vi "Actor Core.vi"(8 "error in":errorcluster, 11 "Timer in":refnum<class "Timer.lvclass">) -> (0 "error out":errorcluster, 3 "Actor out":refnum<class "Actor.lvclass">)   [LabVIEW 2023, in "Timer.lvlib" / "Timer.lvclass"]
doc: "(<B>Filename</B>: Actor Framework.lvlib:Actor.lvclass:Actor Core.vi)\n\nReceives messages to the actor, reacts to them, and initiates any error handling that may shut the actor down.\n\nDescendant classes may override this VI to append parallel tasks for the actor to complete while it handles messages. Overrides use the Call Parent Class Method node."
uses:
  Timer.lvclass
  C:/Program Files/National Instruments/LabVIEW 2023/vi.lib/ActorFramework/Actor/Actor.lvclass
  <vilib>/ActorFramework/Actor/Actor.lvclass
  Timer.lvclass/Timer.ctl
  <vilib>/ActorFramework/Message Enqueuer/Message Priority.ctl
  <vilib>/ActorFramework/Actor/Actor.lvclass/Actor.ctl
  <vilib>/ActorFramework/Message Enqueuer/Message Enqueuer.lvclass/Message Enqueuer.ctl
  <vilib>/ActorFramework/Message Enqueuer/Init from Existing Queue.vi
  <vilib>/ActorFramework/Message Enqueuer/Enqueue.vi
  Timer Messages/Abort Msg/Abort Msg.lvclass
  C:/Program Files/National Instruments/LabVIEW 2023/vi.lib/ActorFramework/Message/Message.lvclass
  <vilib>/ActorFramework/Message Priority Queue/Priority Enqueue.vi
  <vilib>/ActorFramework/Message Enqueuer/Message Enqueuer.lvclass
panel:
  in  "Cancel":bool
  out "Progress":u8(slide) caption="0 s remaining..." scale=0.0..100.0
  out "Stop?":bool=TRUE
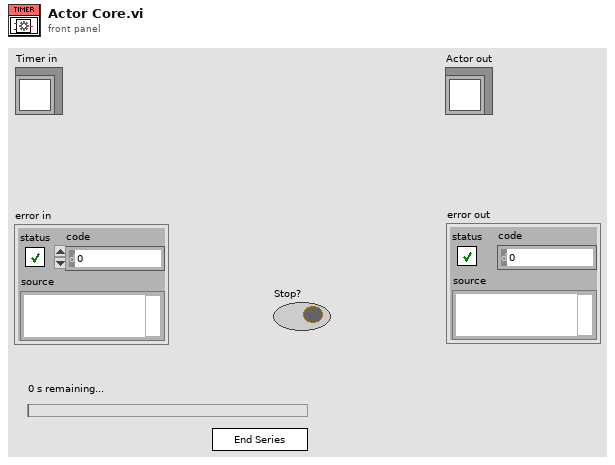
[diagram p1: front panel]
types:
  T1 = enum32{"Invalid", "Standard", "Closed", "Hidden", "Minimized", "Maximized"}
  T2 = typedef "Actor Framework.lvlib/Message Enqueuer.lvclass/Message Priority.ctl" = enum16{"Low", "Normal", "High"}
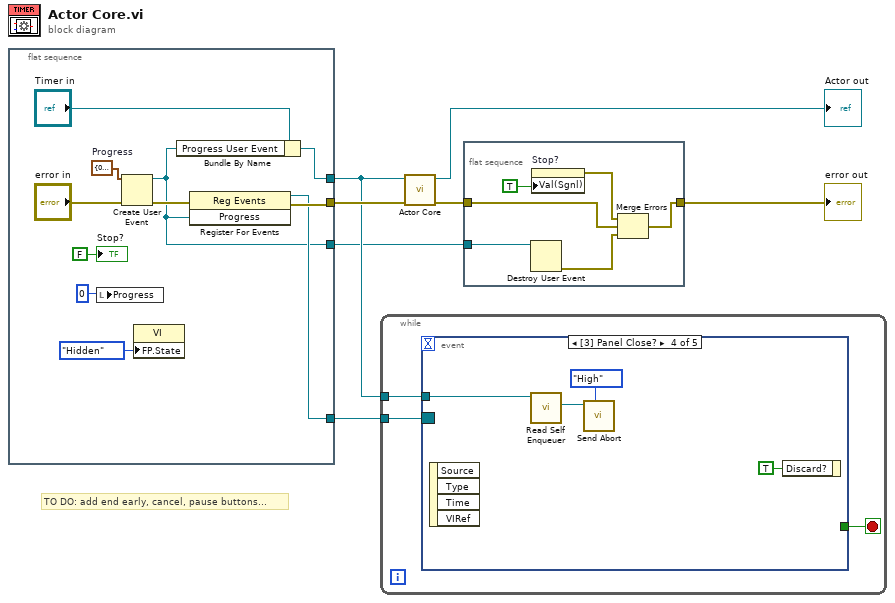
[diagram p0: block diagram]
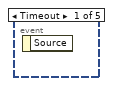
[diagram p2: hidden frame]
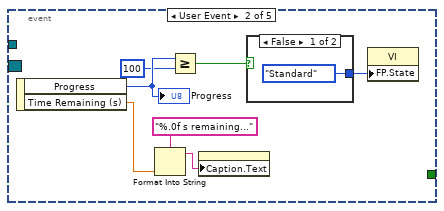
[diagram p3: hidden frame]
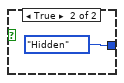
[diagram p4: hidden frame]
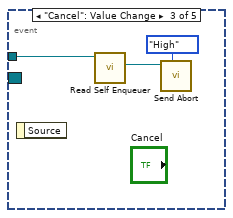
[diagram p5: hidden frame]
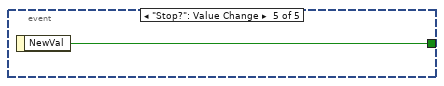
[diagram p6: hidden frame]
diagram:
  # "TO DO: add end early, cancel, pause buttons..."
  n1 = flat-sequence {
    tunnel: [w13] -> w6
    tunnel: [w16] -> w3
    tunnel: [w12] -> w2
    tunnel: [w9] -> w1
    frame #0 {
      w10 = cluster{"Progress":u8, "Time Remaining (s)":dbl} {"Progress"=0, "Time Remaining (s)"=0.0}  # Progress
      n2 = local write "Progress"(u8 0 ("Progress")) -> ()
      n3 = Create User Event(user event datatype=w10, error in="error in") -> (user event=w9:refnum<user-event>, error out=w14:errorcluster)
      n4 = property class="VI"("FP.State"=T1."Hidden" ("Front Panel Window:State")) -> ()  [unwired: 2 in, 2 out]
      n5 = Bundle By Name(cluster="Timer in", "Progress User Event"=w9) -> (w16:refnum<class "Timer.lvclass">)
      n6 = register-events(error in=w14, w9) -> (reference out=w12:refnum<event-registration>, error out=w13:errorcluster)  [unwired: 1 in]
      "Stop?" <- FALSE ("Stop?")
    }
  }
  n7 = while {
    tunnel: w3 -> [w20]
    tunnel: w2 -> [w21]
    stop <- w19 stop-if-true
    n8 = event shown="[3] Panel Close?" {
      selector: w21 -> [_ _ _ _ _]
      dyn-events: _ -> [_ _ _ _ _]
      timeout: _ -> [_ _ _ _ _]
      tunnel: w20 -> [_ _ w33 w36 _]
      tunnel: [_ _ _ _ w38] -> w19
      event Timeout {
        n9 = event-data() -> ()  [unwired: 1 in, 1 out]
      }
      event User Event {
        n10 = event-data() -> ("Progress"=w25:u8, "Time Remaining (s)"=w26:dbl)  [unwired: 1 in]
        "Progress" <- w25
        n11 = Format Into String(format string="%.0f s remaining...", w26) -> (resulting string=w28:string)  [unwired: 2 in, 1 out]
        n12 = Greater Or Equal?(x=w25, y=u8 100) -> (x >= y?=w23:bool)
        n13 = property on="Progress" class="Slide (strict)"("Caption.Text"=w28) -> ()  [unwired: 2 in, 2 out]
        n14 = case shown="False" w23 {
          tunnel: [T1."Standard" ("Front Panel Window:State") T1."Hidden" ("Front Panel Window:State")] -> w22
          frame False {
          }
          frame True {
          }
        }
        n15 = property class="VI"("FP.State"=w22) -> ()  [unwired: 2 in, 2 out]
      }
      event "Cancel": Value Change {
        n16 = event-data() -> ()  [unwired: 1 in, 1 out]
        n17 = call <vilib>:"Read Self Enqueuer.vi"("Actor"=w33) -> ("Self Enqueuer"=w32:refnum<class "Message Enqueuer.lvclass">)  [unwired: 10 in]
        n18 = call "Send Abort.vi"("Message Priority (Normal)"=Message_Priority."High", "Message Enqueuer"=w32) -> ()  [unwired: 8 in, 2 out]
      }
      event Panel Close? {
        n19 = event-data() -> ()  [unwired: 1 in, 4 out]
        n20 = call <vilib>:"Read Self Enqueuer.vi"("Actor"=w36) -> ("Self Enqueuer"=w35:refnum<class "Message Enqueuer.lvclass">)  [unwired: 10 in]
        n21 = call "Send Abort.vi"("Message Priority (Normal)"=Message_Priority."High", "Message Enqueuer"=w35) -> ()  [unwired: 8 in, 2 out]
        n22 = event-data("Discard?"=TRUE) -> ()  [unwired: 1 in, 1 out]
      }
      event "Stop?": Value Change {
        n23 = event-data() -> ("NewVal"=w38:bool)  [unwired: 1 in]
      }
    }
  }
  n24 = call-parent "Actor Core.vi"("error in"=w6, "Actor in"=w3) -> ("error out"=w5:errorcluster, "Actor out"=→"Actor out":refnum<class "Actor.lvclass">)  [unwired: 8 in]
  n25 = flat-sequence {
    tunnel: w5 -> [w41]
    tunnel: [w39] -> w4
    tunnel: w1 -> [w43]
    frame #0 {
      n26 = Destroy User Event(user event=w43) -> (error out=w40:errorcluster)  [unwired: 1 in]
      n27 = property on="Stop?" class="Bool (strict)"("Val(Sgnl)"=TRUE ("Stop?")) -> (error out=w42:errorcluster)  [unwired: 2 in, 1 out]
      n28 = Merge Errors(w42, w41, w40) -> (w39:errorcluster)
    }
  }
  "error out" <- w4
